vi "Get Shape.vi"(11 "Drawable in":refnum<class "Drawable.lvclass">) -> (1 "Color":u32(colorbox), 2 "Coordinates":cluster{"X":i32, "Y":i32}[](array[cluster]), 3 "Drawable out":refnum<class "Drawable.lvclass">)   [LabVIEW 2020, in "Drawable.lvclass"]
uses:
  Drawable.lvclass
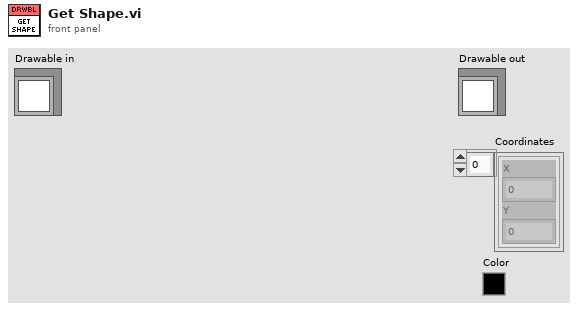
[diagram p1: front panel]
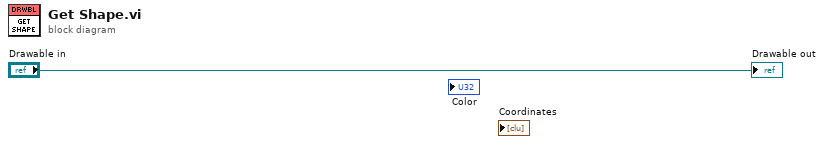
[diagram p0: block diagram]
diagram:
  "Drawable out" <- "Drawable in"
